vi "Pacemaker ASIC Test_Search Value.vi"(10 "y":dbl, 11 "data":dbl[](array[numeric])) -> (3 "x":i32)   [LabVIEW 2016]
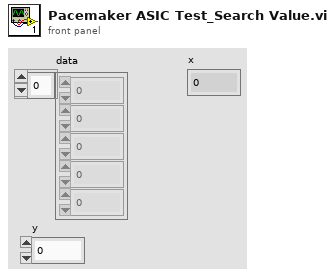
[diagram p1: front panel]
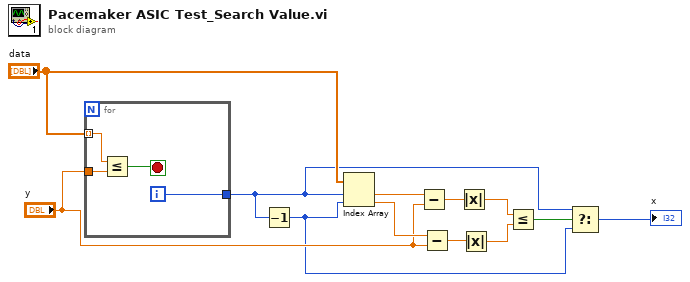
[diagram p0: block diagram]
diagram:
  n1 = for {
    tunnel: "data" -> [w16] mode=indexing
    tunnel: "y" -> [w15]
    tunnel: [w13] -> w3
    i -> [w13]
    stop <- w14 stop-if-true
    n2 = Less Or Equal?(x=w16, y=w15) -> (x <= y?=w14:bool)
  }
  n3 = Decrement(x=w3) -> (x-1=w2:i32)
  n4 = Index Array(array="data", index #1=w3, index #2=w2) -> (element #1=w11:dbl, element #2=w10:dbl)
  n5 = Subtract(x=w11, y="y") -> (x-y=w8:dbl)
  n6 = Subtract(x=w10, y="y") -> (x-y=w7:dbl)
  n7 = Absolute Value(x=w8) -> (abs(x)=w6:dbl)
  n8 = Absolute Value(x=w7) -> (abs(x)=w5:dbl)
  n9 = Less Or Equal?(x=w6, y=w5) -> (x <= y?=w4:bool)
  n10 = Select(t=w3, s=w4, f=w2) -> (s? t:f=→"x":i32)
